vi "curvness detection.vi"(0 "2D curv array in":dbl[][](array[numeric]), 1 "array sensor in":dbl[](array[numeric]), 2 "avg wind1":i32, 3 "min level thr":dbl[](array[numeric]), 4 "coloumn count":bool=TRUE, 5 "curv Array":dbl[](array[numeric]), 6 "col count":i32, 7 "error in (no error)":errorcluster) -> (14 "2D curv array Out":dbl[][](array[numeric]), 17 "distance array":dbl[](array[numeric]), 18 "curv Array out":dbl[](array[numeric]), 19 "error out":errorcluster)   [LabVIEW 2019]
uses:
  <vilib>/Analysis/baseanly.llb/Multimode.vi
  <vilib>/measure/mamon.llb/Trigger Detection for 1 Channel.vi
  <vilib>/measure/NI_MAPro.lvlib
  <vilib>/Analysis/NI_AALBase.lvlib
panel:
  out "Numeric":dbl
  out "output array":dbl[](array[numeric])
  out "2D curv array in 2":dbl[][](array[numeric])
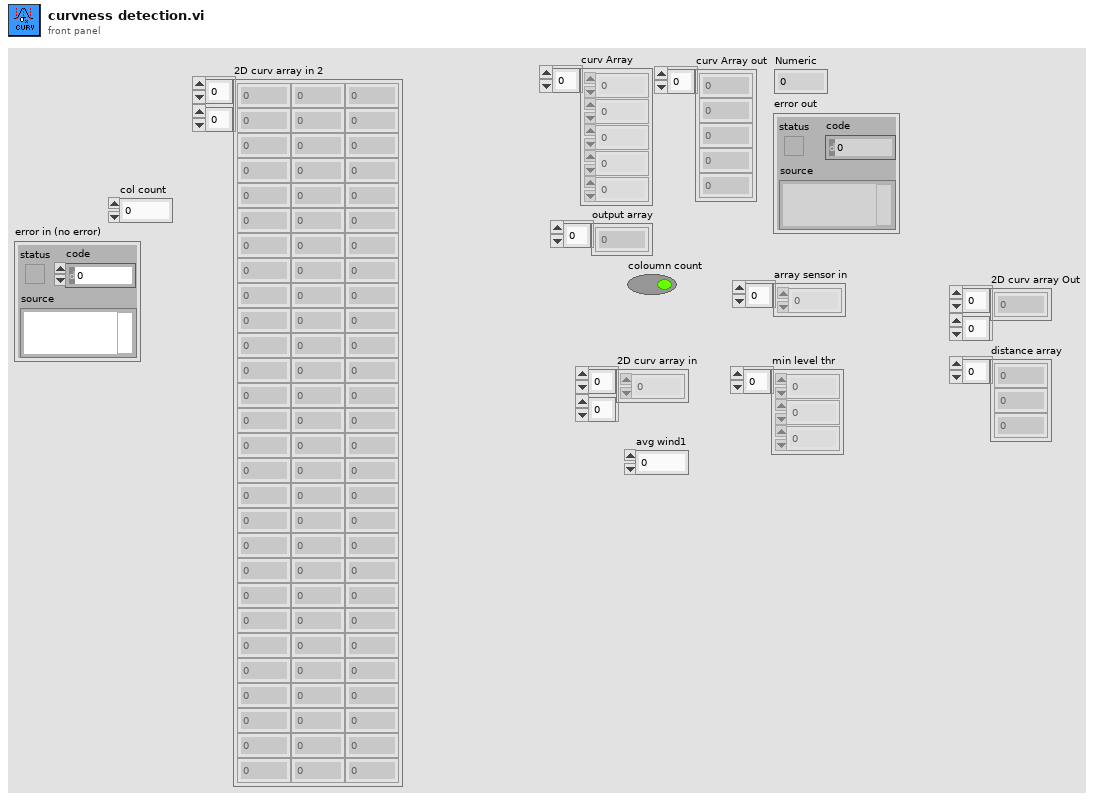
[diagram p1: front panel]
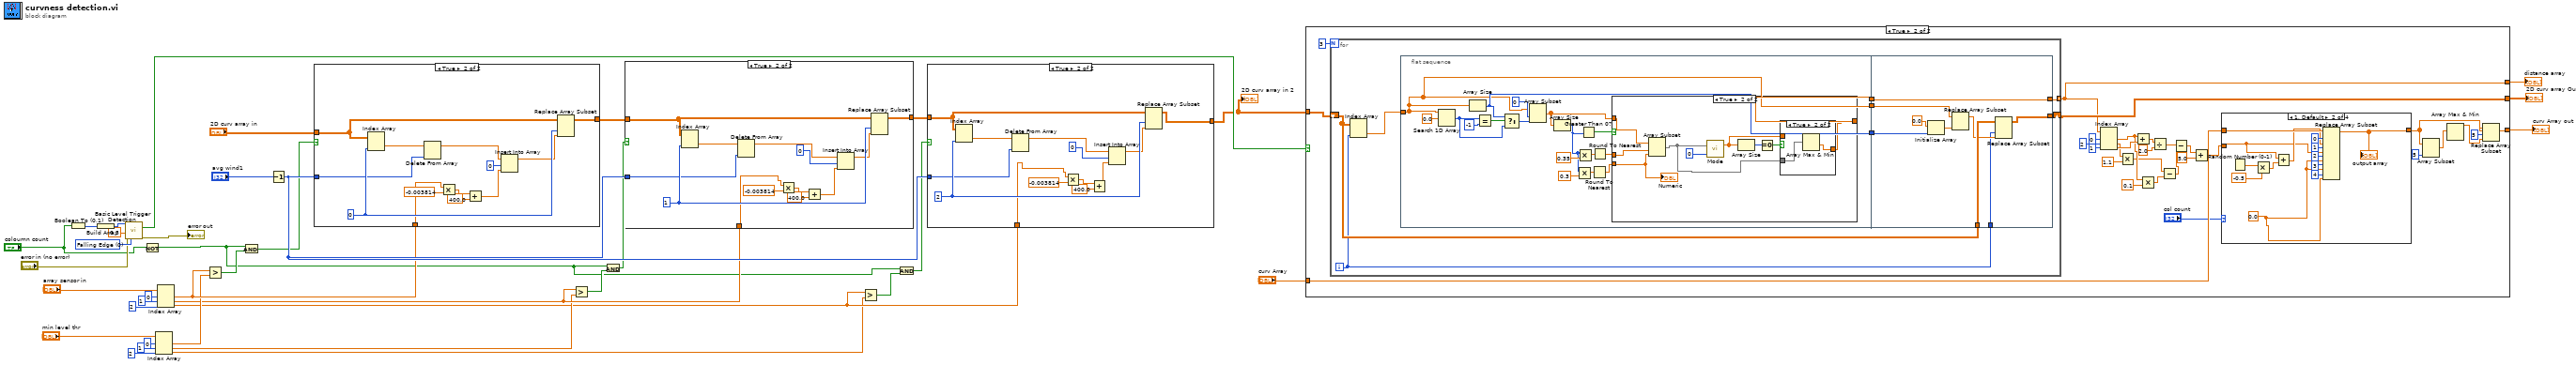
[diagram p0: block diagram]
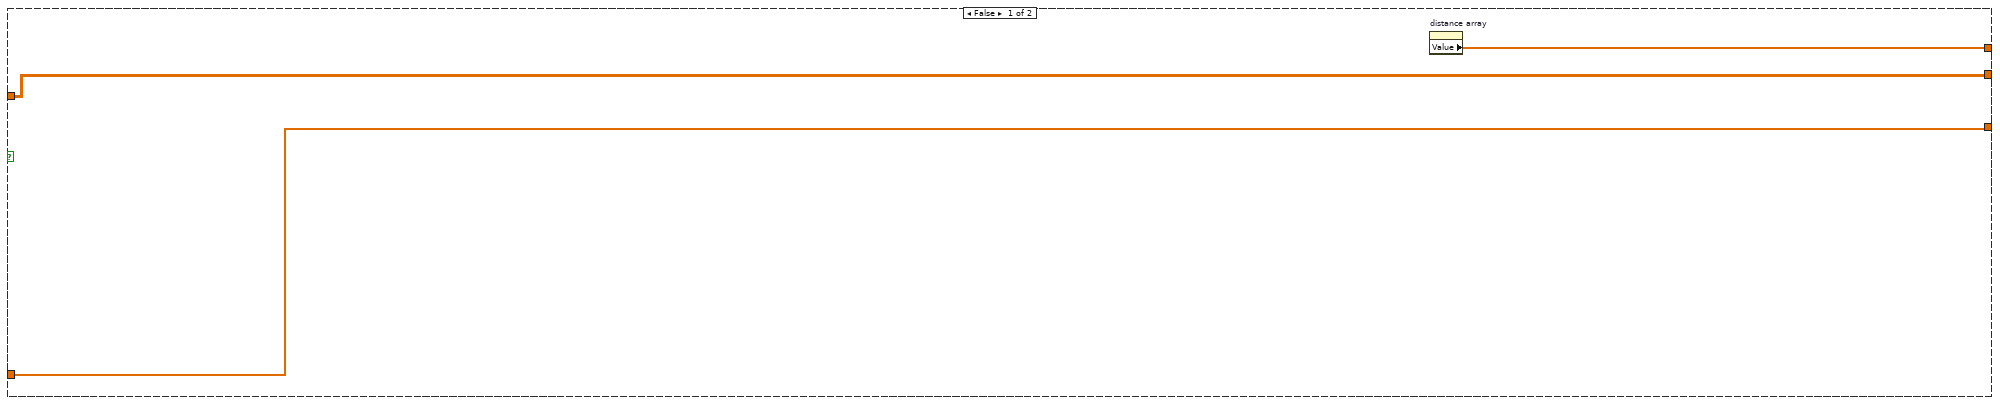
[diagram p2: hidden frame]
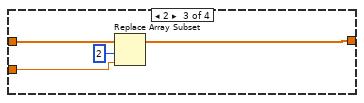
[diagram p4: hidden frame]
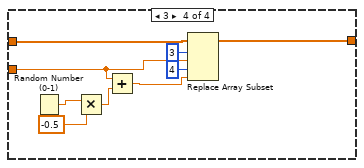
[diagram p5: hidden frame]
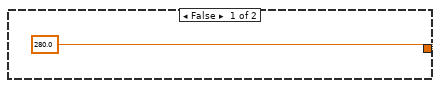
[diagram p6: hidden frame]
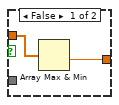
[diagram p7: hidden frame]
diagram:
  w5 = u16 0 items=["Falling Edge", "Rising Edge"] ("trigger slope")
  n1 = Boolean To (0,1)(Boolean="coloumn count") -> (0, 1=w12:i16)
  n2 = Build Array(w12) -> (w11:i16[])
  n3 = call-poly <vilib>:"Basic Level Trigger Detection.vi"("signal in"=w11, "level"=0.5, "error in (no error)"="error in (no error)", "trigger slope"=w5) -> ("trigger detected?"=w9:bool, "error out"=→"error out":errorcluster)  [unwired: 9 in, 1 out]
  n4 = Not(x="coloumn count") -> (.not. x?=w1:bool)
  n5 = Index Array(array="min level thr", index #1=0 ("index"), index #2=1 ("index"), index #3=2 ("index")) -> (element #1=w25:dbl, element #2=w20:dbl, element #3=w17:dbl)
  n6 = Index Array(array="array sensor in", index #1=0 ("index"), index #2=1 ("index"), index #3=2 ("index")) -> (element #1=w30:dbl, element #2=w21:dbl, element #3=w18:dbl)
  n7 = Greater?(x=w30, y=w25) -> (0:w24:bool)
  n8 = And(x=w1, y=w24) -> (x .and. y?=w23:bool)
  n9 = Decrement(x="avg wind1") -> (x-1=w35:i32)
  n10 = case shown="True" w23 {
    tunnel: "2D curv array in" -> [w40 w50]
    tunnel: [w40 w48] -> w38
    tunnel: w35 -> [_ w46]
    tunnel: w30 -> [_ w45]
    frame False {
    }
    frame True {
      w49 = 0 ("col sel")
      n11 = Index Array "Index Array"(array=w50, index (col)=w49) -> (element=w52:dbl[])  [unwired: 1 in]
      n12 = Delete From Array "Delete From Array"(array=w52, index=w46) -> (array with subset deleted=w51:dbl[])  [unwired: 1 in, 1 out]
      n13 = Multiply(x=w45, y=-0.003814) -> (x*y=w43:dbl)
      n14 = Add(x=w43, y=400.0) -> (x+y=w41:dbl)
      n15 = Insert Into Array "Insert Into Array"(array=w51, index=0, new element=w41) -> (w47:dbl[])
      n16 = Replace Array Subset "Replace Array Subset"(array=w50, new element=w47, index (col)=w49) -> (w48:dbl[][])  [unwired: 1 in]
    }
  }
  n17 = Greater?(x=w21, y=w20) -> (0:w22:bool)
  n18 = And(x=w1, y=w22) -> (x .and. y?=w16:bool)
  n19 = case shown="True" w16 {
    tunnel: w38 -> [w54 w63]
    tunnel: [w54 w62] -> w37
    tunnel: w35 -> [_ w60]
    tunnel: w21 -> [_ w56]
    frame False {
    }
    frame True {
      w67 = 1 ("col sel 2")
      n20 = Index Array "Index Array"(array=w63, index (col)=w67) -> (element=w65:dbl[])  [unwired: 1 in]
      n21 = Delete From Array "Delete From Array"(array=w65, index=w60) -> (array with subset deleted=w66:dbl[])  [unwired: 1 in, 1 out]
      n22 = Multiply(x=w56, y=-0.003814) -> (x*y=w58:dbl)
      n23 = Add(x=w58, y=400.0) -> (x+y=w55:dbl)
      n24 = Insert Into Array "Insert Into Array"(array=w66, index=0, new element=w55) -> (w61:dbl[])
      n25 = Replace Array Subset "Replace Array Subset"(array=w63, new element=w61, index (col)=w67) -> (w62:dbl[][])  [unwired: 1 in]
    }
  }
  n26 = Greater?(x=w18, y=w17) -> (0:w19:bool)
  n27 = And(x=w1, y=w19) -> (x .and. y?=w15:bool)
  n28 = case shown="True" w15 {
    tunnel: w37 -> [w68 w77]
    tunnel: [w68 w76] -> w8
    tunnel: w35 -> [_ w74]
    tunnel: w18 -> [_ w70]
    frame False {
    }
    frame True {
      w78 = 2 ("col sel 3")
      n29 = Index Array "Index Array"(array=w77, index (col)=w78) -> (element=w80:dbl[])  [unwired: 1 in]
      n30 = Delete From Array "Delete From Array"(array=w80, index=w74) -> (array with subset deleted=w79:dbl[])  [unwired: 1 in, 1 out]
      n31 = Multiply(x=w70, y=-0.003814) -> (x*y=w72:dbl)
      n32 = Add(x=w72, y=400.0) -> (x+y=w69:dbl)
      n33 = Insert Into Array "Insert Into Array"(array=w79, index=0, new element=w69) -> (w75:dbl[])
      n34 = Replace Array Subset "Replace Array Subset"(array=w77, new element=w75, index (col)=w78) -> (w76:dbl[][])  [unwired: 1 in]
    }
  }
  "2D curv array in 2" <- w8
  n35 = case shown="True" w9 {
    tunnel: w8 -> [w84 w113]
    tunnel: [w84 w111] -> w14
    tunnel: [w83 w110] -> w13
    tunnel: "curv Array" -> [w82 w104]
    tunnel: [w82 w100] -> w6
    frame False {
      n36 = property on="distance array" class="Arr (strict)"() -> ("Value"=w83:dbl[])  [unwired: 2 in, 2 out]
    }
    frame True {
      n37 = for {
        N: 3 -> [_]
        tunnel: [w145] -> w110 mode=indexing
        shift-right: [w141] -> w111
        shift-left: w113 -> [w143]
        i -> [w142]
        n38 = Index Array(array=w143, index (col)=w142) -> (element=w144:dbl[])  [unwired: 1 in]
        n39 = flat-sequence {
          tunnel: w144 -> [w156]
          tunnel: [w161] -> w148
          tunnel: [w156] -> w147
          tunnel: [w158] -> w146
          tunnel: w148 -> [w188]
          tunnel: w147 -> [w187]
          tunnel: [w185] -> w145
          tunnel: w146 -> [w185]
          tunnel: w143 -> [w184]
          tunnel: w142 -> [w182]
          tunnel: [w181] -> w141
          frame #0 {
            n40 = Search 1D Array(1D array=w156, element=0.0) -> (index of element=w160:i32)  [unwired: 1 in]
            n41 = Array Size(array=w156) -> (size(s)=w161:i32)
            n42 = Equal?(x=w160, y=-1) -> (x = y?=w163:bool)
            n43 = Select(t=w161, s=w163, f=w160) -> (s? t:f=w162:i32)
            n44 = Array Subset(array=w156, index=0, length=w162) -> (w159:dbl[])
            n45 = Array Size(array=w159) -> (size(s)=w150:i32)
            n46 = Multiply(x=w150, y=0.3) -> (x*y=w153:dbl)
            n47 = Multiply(x=w150, y=0.35) -> (x*y=w155:dbl)
            n48 = Greater Than 0?(x=w150) -> (x > 0?=w157:bool)
            n49 = Round To Nearest(number=w153) -> (nearest integer value=w149:dbl)
            n50 = Round To Nearest(number=w155) -> (nearest integer value=w154:dbl)
            n51 = case shown="True" w157 {
              tunnel: w159 -> [_ w176]
              tunnel: [280.0 w173] -> w158
              tunnel: w154 -> [_ w175]
              tunnel: w149 -> [_ w174]
              frame False {
              }
              frame True {
                n52 = Array Subset(array=w176, index=w175, length=w174) -> (w168:dbl[])
                n53 = call-poly <vilib>:"Mode.vi"("intervals"=0, "X"=w168) -> ("Modes"=w169:dbl[])  [unwired: 1 out]
                n54 = Array Size(array=w169) -> (size(s)=w170:i32)
                n55 = Equal To 0?(x=w170) -> (x = 0?=w171:bool)
                n56 = case shown="True" w171 {
                  tunnel: [w178 w179] -> w173
                  tunnel: w169 -> [w177 _]
                  tunnel: w168 -> [_ w180]
                  frame False {
                    n57 = Array Max & Min(array=w177) -> (min value=w178:dbl)  [unwired: 3 out]
                  }
                  frame True {
                    n58 = Array Max & Min(array=w180) -> (min value=w179:dbl)  [unwired: 3 out]
                  }
                }
                "Numeric" <- w174
              }
            }
          }
          frame #1 {
            n59 = Initialize Array(0.0 ("element"), w188) -> (w186:dbl[])
            n60 = Replace Array Subset(array=w187, new element=w186) -> (w183:dbl[])  [unwired: 1 in]
            n61 = Replace Array Subset "Replace Array Subset"(array=w184, new element=w183, index (col)=w182) -> (w181:dbl[][])  [unwired: 1 in]
          }
        }
      }
      n62 = Index Array(array=w110, index #1=0 ("index"), index #2=2 ("index"), index #3=1 ("index")) -> (element #1=w92:dbl, element #2=w94:dbl, element #3=w106:dbl)
      n63 = Multiply(x=w94, y=1.1) -> (x*y=w89:dbl)
      n64 = Add(x=w92, y=w106) -> (x+y=w105:dbl)
      n65 = Multiply(x=w92, y=0.1) -> (x*y=w90:dbl)
      n66 = Divide(x=w105, y=2.0) -> (x/y=w96:dbl)
      n67 = Subtract(x=w89, y=w90) -> (x-y=w88:dbl)
      n68 = Subtract(x=w96, y=w88) -> (x-y=w87:dbl)
      n69 = Add(x=w87, y=5.0) -> (x+y=w85:dbl)
      n70 = case shown="1, Default" "col count" {
        tunnel: w104 -> [w114 w127 w131 w139]
        tunnel: w85 -> [_ w115 w129 w133]
        tunnel: [w114 w120 w128 w137] -> w97
        frame 0 {
        }
        frame 1, Default {
          w121 = 0.0 ("new element/subarray")
          n71 = Random Number (0-1)() -> (number: 0 to 1=w119:dbl)
          n72 = Multiply(x=w119, y=-0.5) -> (x*y=w117:dbl)
          n73 = Add(x=w115, y=w117) -> (x+y=w116:dbl)
          n74 = Replace Array Subset(array=w127, new element #1=w116, index #1=0 ("index"), new element #2=w115, index #2=1 ("index"), new element #3=w121, index #3=2 ("index"), new element #4=w121, index #4=3 ("index"), new element #5=w121, index #5=4 ("index")) -> (w120:dbl[])
          "output array" <- w120
        }
        frame 2 {
          n75 = Replace Array Subset(array=w131, new element=w129, index=2) -> (w128:dbl[])
        }
        frame 3 {
          n76 = Random Number (0-1)() -> (number: 0 to 1=w136:dbl)
          n77 = Multiply(x=w136, y=-0.5) -> (x*y=w134:dbl)
          n78 = Add(x=w133, y=w134) -> (x+y=w132:dbl)
          n79 = Replace Array Subset(array=w139, new element #1=w133, index #1=3 ("index"), new element #2=w132, index #2=4 ("index")) -> (w137:dbl[])
        }
      }
      n80 = Array Subset(array=w97, length=5) -> (w98:dbl[])  [unwired: 1 in]
      n81 = Array Max & Min(array=w98) -> (max value=w101:dbl)  [unwired: 3 out]
      n82 = Replace Array Subset(array=w97, new element=w101, index=5) -> (w100:dbl[])
    }
  }
  "2D curv array Out" <- w14
  "distance array" <- w13
  "curv Array out" <- w6
